vi "Request Grabber State.vi"(8 "error in (no error)":errorcluster, 9 "Requestor Queue":refnum<class "Message Enqueuer.lvclass">, 10 "Grabber.lvlib:Current Grabber State Msg.lvclass":refnum<class "Current Grabber State Msg.lvclass">, 11 "Grabber in":refnum<class "Grabber.lvclass">) -> (0 "error out":errorcluster, 3 "Grabber out":refnum<class "Grabber.lvclass">)   [LabVIEW 2014, in "Grabber.lvlib" / "Grabber.lvclass"]
uses:
  Grabber.lvclass
  <vilib>/ActorFramework/Message Enqueuer/Message Enqueuer.lvclass
  Grabber Messages/Current Grabber State Msg/Current Grabber State Msg.lvclass
  Grabber.lvclass/Grabber.ctl
  Grabber Messages/Current Grabber State Msg/Current Grabber State Msg.lvclass/Current Grabber State Msg.ctl
  <vilib>/ActorFramework/Message Enqueuer/Message Enqueuer.lvclass/Message Enqueuer.ctl
  <vilib>/ActorFramework/Message Enqueuer/Enqueue.vi
  <vilib>/ActorFramework/Message Priority Queue/Priority Enqueue.vi
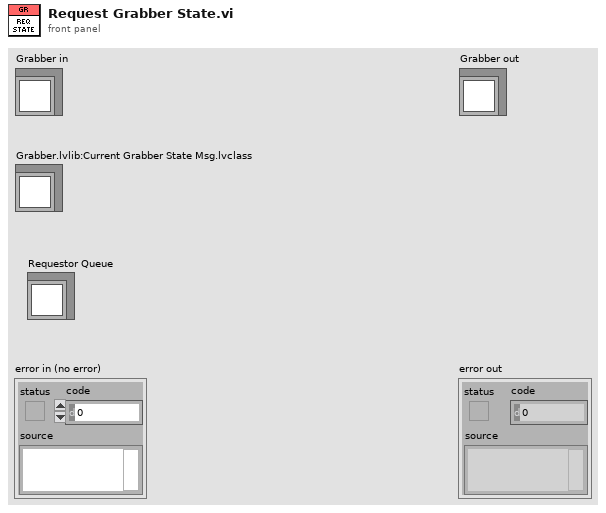
[diagram p1: front panel]
types:
  T1 = typedef "Grabber.lvlib/Grabber.lvclass/Grabber State.ctl" = cluster{"Arms Closed":bool, "Left Wheel Power":dbl, "Right Wheel Power":dbl}
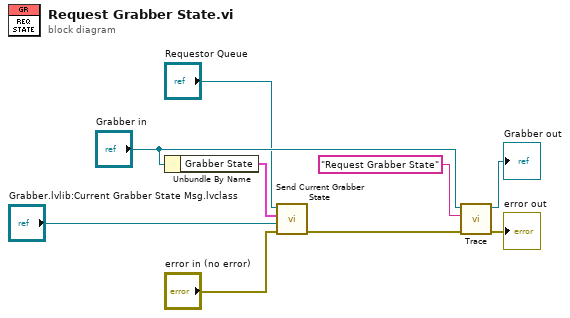
[diagram p0: block diagram]
diagram:
  n1 = Unbundle By Name("Grabber in") -> ("Grabber State"=w5:T1)
  n2 = call "Send Current Grabber State.vi"("error in (no error)"="error in (no error)", "Grabber.lvlib:Current Grabber State Msg.lvclass"="Grabber.lvlib:Current Grabber State Msg.lvclass", "Grabber State"=w5, "Message Enqueuer"="Requestor Queue") -> ("error out"=w2:errorcluster)  [unwired: 6 in, 1 out]
  n3 = call-dynamic "Trace.vi"("error in (no error)"=w2, "System Action"="Request Grabber State", "System Actor in"="Grabber in") -> ("error out"=→"error out":errorcluster, "System Actor out"=→"Grabber out":refnum<class "Grabber.lvclass">)  [unwired: 7 in]
